vi "niRFUtil WFM Unwrap Phase (complex array).vi"(0 "Complex Vectors":T2 format="%.2f") -> (4 "Magnitude":T1 min=0 max=127 format="%.2f", 6 "Unwrapped Phase (rad)":T1 min=0 max=127 format="%.2f")   [LabVIEW 2015, in "niRFUtil.lvlib"]
uses:
  niRFUtil.lvlib
  Includes/niRFUtil INC Complex Array.ctl
  Includes/niRFUtil INC Real Array.ctl
  Measurements/niRFUtil MEAS Mean (real array).vi
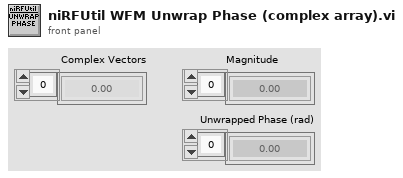
[diagram p1: front panel]
types:
  T1 = typedef "niRFUtil.lvlib/niRFUtil INC Real Array.ctl" = sgl[]
  T2 = typedef "niRFUtil.lvlib/niRFUtil INC Complex Array.ctl" = csg[]
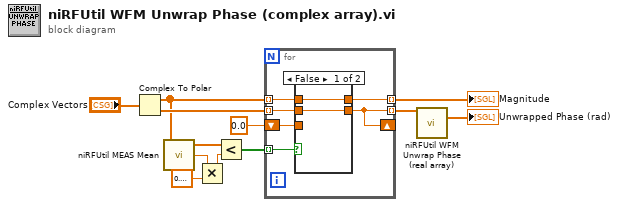
[diagram p0: block diagram]
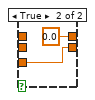
[diagram p2: hidden frame]
diagram:
  n1 = Complex To Polar(r * e^(i*theta)="Complex Vectors") -> (r=w5:sgl[], theta=w7:sgl[])
  n2 = call-poly "niRFUtil MEAS Mean.vi"("Real Array"=w5) -> ("Mean"=w9:sgl)  [unwired: 14 in]
  n3 = Multiply(x=w9, y=sgl 0.1) -> (x*y=w11:sgl)
  n4 = Less?(x=w5, y=w11) -> (x < y?=w8:bool[])
  n5 = for {
    tunnel: w7 -> [w16] mode=indexing
    tunnel: w8 -> [w17] mode=indexing
    tunnel: [w12] -> w2 mode=indexing
    shift-right: [w12] -> _
    shift-left: sgl 0.0 -> [w13]
    tunnel: w5 -> [w15] mode=indexing
    tunnel: [w14] -> w3 mode=indexing
    n6 = case shown="False" w17 {
      tunnel: w16 -> [w19 _]
      tunnel: [w19 w21] -> w12
      tunnel: w13 -> [_ w21]
      tunnel: w15 -> [w18 _]
      tunnel: [w18 sgl 0.0 ("Numeric")] -> w14
      frame False {
      }
      frame True {
      }
    }
  }
  "Magnitude" <- w3
  n7 = call "niRFUtil WFM Unwrap Phase (real array).vi"("Phase In (rad)"=w2) -> ("Phase Out (rad)"=→"Unwrapped Phase (rad)":T1)  [unwired: 14 in]
